vi "Manual Mode.vi"(0 "potent":dbl, 1 "Shooter":dbl, 2 "climb":bool, 3 "Button 1":bool, 5 "manual":bool) -> ()   [LabVIEW 2012]
uses:
  <vilib>/Rock Robotics/WPI/Solenoid/WPI_SolenoidValue.ctl
  <vilib>/Rock Robotics/WPI/Solenoid/WPI_SolenoidSetEnum.vi
  <vilib>/Rock Robotics/WPI/Joystick/WPI_JoystickGetSetRefNum.vi
  <vilib>/Rock Robotics/WPI/RobotDrive/WPI_RobotDriveArcadeDrive_Standard(NoSaturation).vi
  <vilib>/Rock Robotics/WPI/RobotDrive/WPI_RobotDriveGetSetRefNum.vi
panel:
  in  "Kick?":bool
  in  "Select":dbl(slide)=2.502610966057441 scale=0.3..4.1
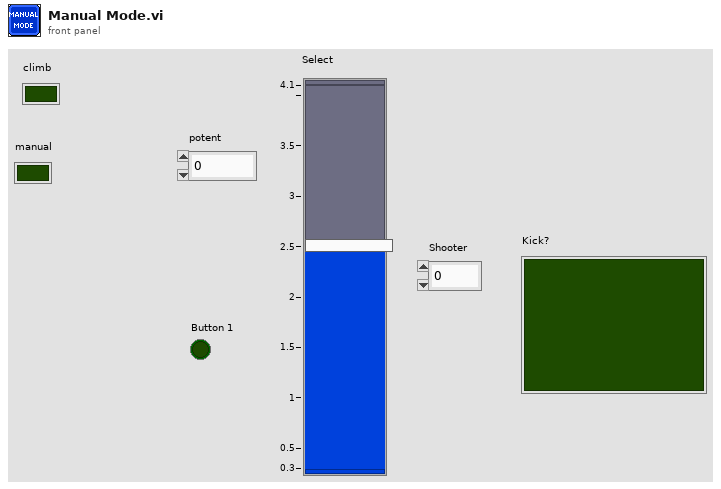
[diagram p1: front panel]
types:
  T1 = typedef "WPI_SolenoidValue.ctl" = enum16{"Off", "On", "Forward", "Reverse"}
  T2 = typedef "WPI_JoystickDevRef.ctl" = cluster{"Device":T3}
  T3 = typedef "WPI_JoystickDeviceEnum.ctl" = enum16{"USB 1", "USB 2", "USB 3", "USB 4", "Kinect 1", "Kinect 2"}
  T4 = typedef "WPI_JoystickButtonState.ctl" = cluster{"Button 1":bool, "Button 2":bool, "Button 3":bool, "Button 4":bool, "Button 5":bool, "Button 6":bool, "Button 7":bool, "Button 8":bool, "Button 9":bool, "Button 10":bool, "Button 11":bool, "Button 12":bool}
  T5 = typedef "WPI_MotorControlDeviceRef.ctl" = cluster{"DeviceStatus":errorcluster, "Type":enum16{"PWM", "CAN"}, "PWM":cluster{"Digital Module":T6, "PWM Channel":T7, "DeadBand":T8}, "CAN":cluster{"Device Number":u8, "Control Mode":T9, "Semaphore":T10, "Max Vout":dbl}, "Invert":bool, "TransformRef":T11, "InvTransformRef":T11}
  T6 = typedef "FPGA_TypedefDigitalModule.ctl" = enum16{"Digital Module 1", "Digital Module 2"}
  T7 = typedef "FPGA_DIOPWMChannel.ctl" = enum8{"PWM 1", "PWM 2", "PWM 3", "PWM 4", "PWM 5", "PWM 6", "PWM 7", "PWM 8", "PWM 9", "PWM 10", "Invalid"}
  T8 = typedef "WPI_PWMDeadband.ctl" = cluster{"Name":string, "maxPositivePwm":i32, "minPositivePwm":i32, "centerPwm":i32, "maxNegativePwm":i32, "minNegativePwm":i32, "angularRange":u16}
  T9 = typedef "WPI_CANJaguar_ControlMode.ctl" = enum8{"Percent VBus", "Current", "Speed", "Position", "Voltage"}
  T10 = typedef "Semaphore RefNum" = refnum<k1>
  T11 = typedef "WPI_PWMTransform_ConPane.ctl" = refnum<vi>
  T12 = typedef "WPI_SolenoidDevRef.ctl" = cluster{"DevStatus":errorcluster, "Solenoid Module":T13, "Forward Solenoid Channel":T14, "Reverse Solenoid Channel":T14}
  T13 = typedef "FPGA_TypedefSolenoidModule.ctl" = enum16{"Solenoid Module 1", "Solenoid Module 2"}
  T14 = typedef "WPI_SolenoidChannel.ctl" = enum8{"Solenoid 1", "Solenoid 2", "Solenoid 3", "Solenoid 4", "Solenoid 5", "Solenoid 6", "Solenoid 7", "Solenoid 8", "Invalid"}
  T15 = typedef "WPI_RobotDriveDevRef.ctl" = cluster{"DevStatus":errorcluster, "Motors[]":T5[], "Square Inputs":bool, "Max Output":dbl, "Isochronous":bool}
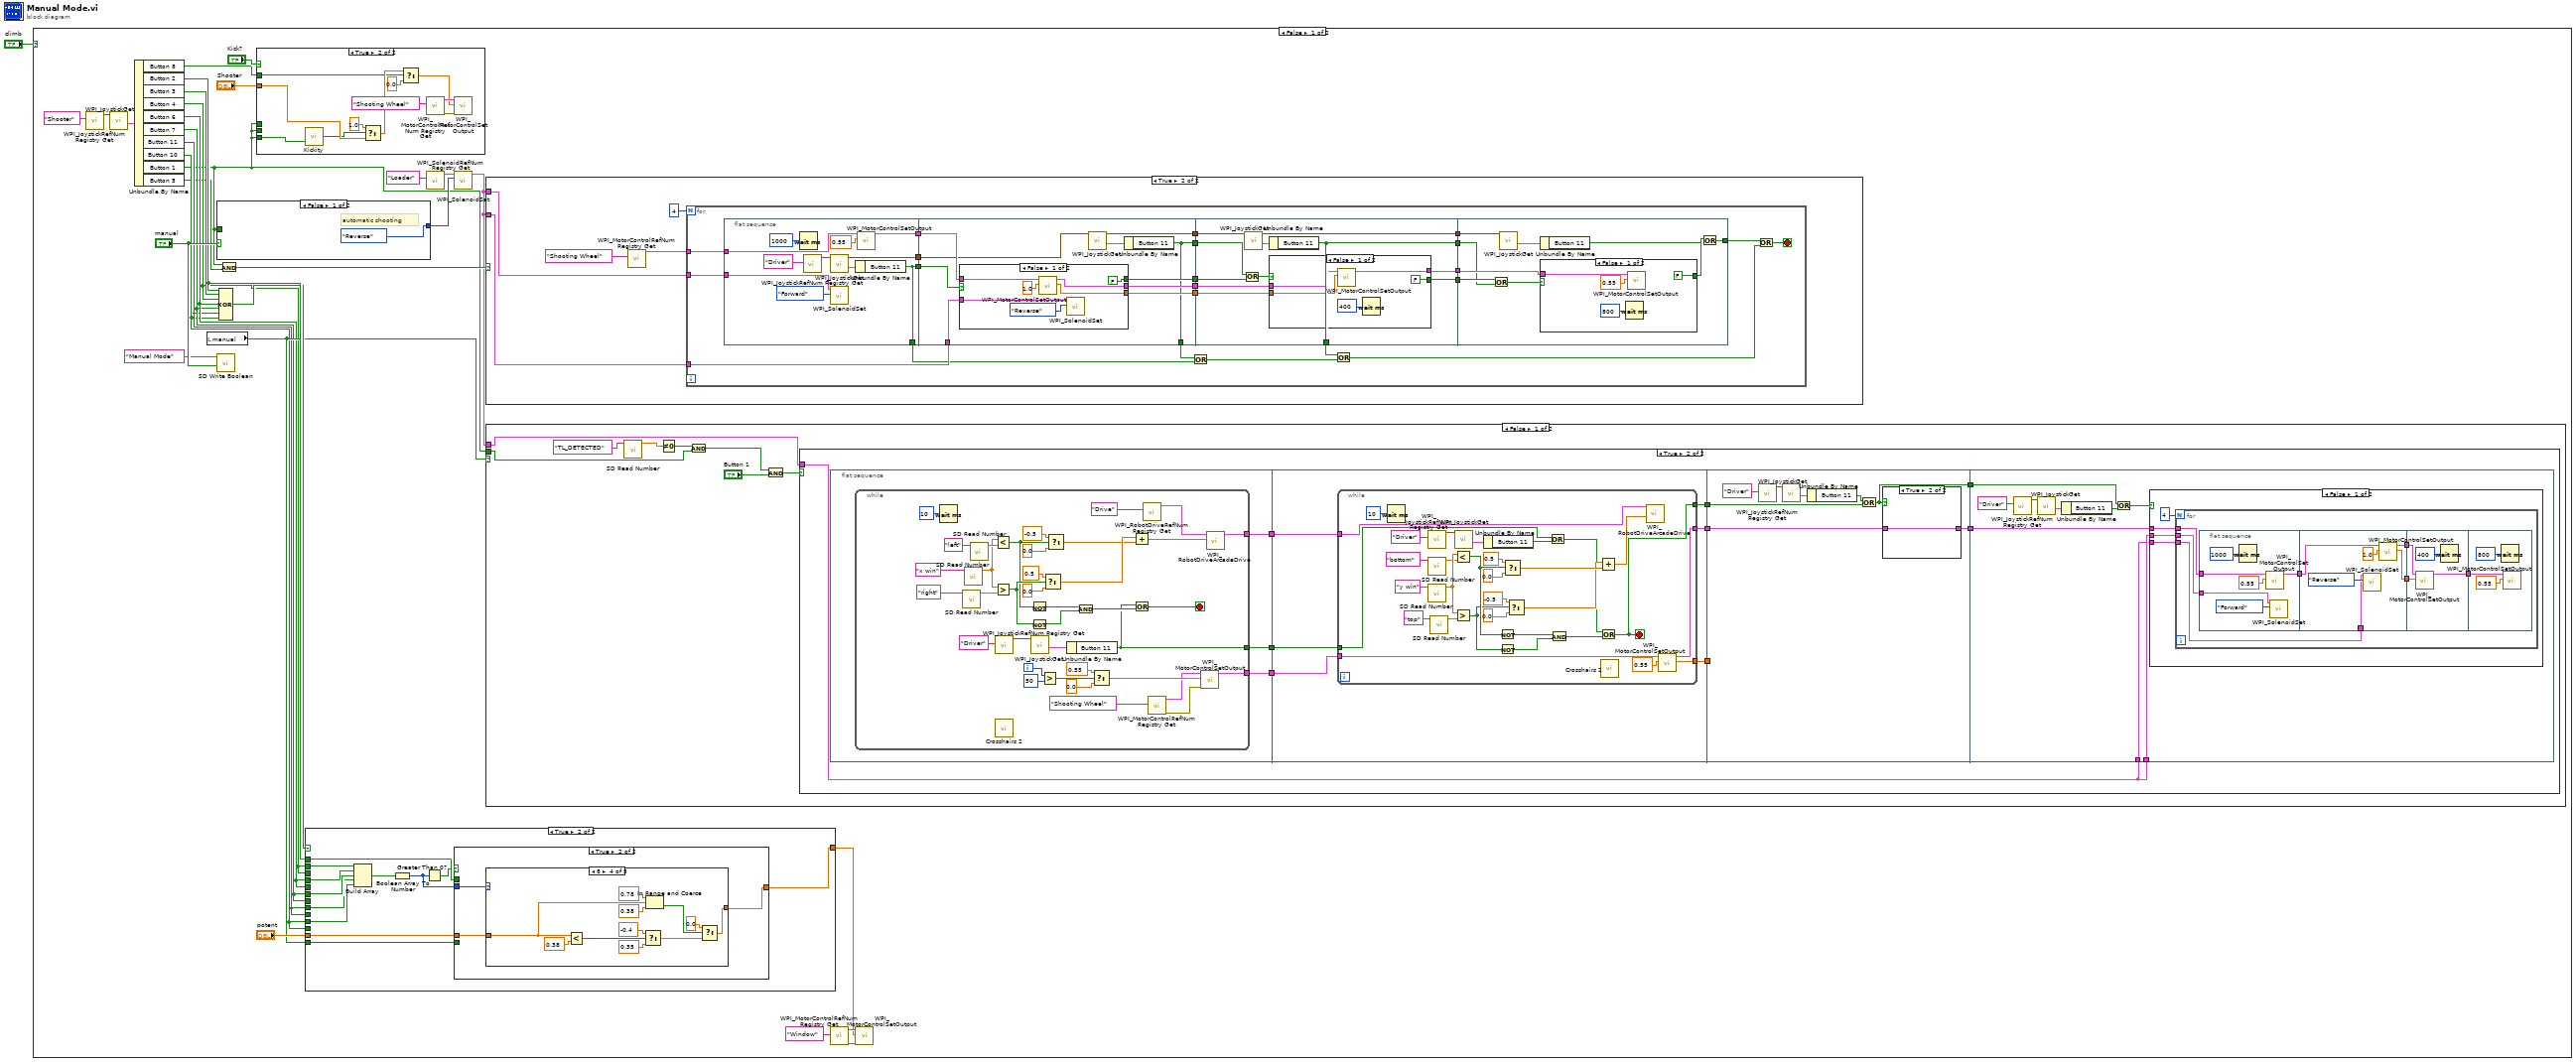
[diagram p0: block diagram]
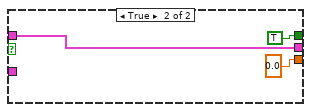
[diagram p3: hidden frame]
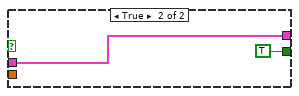
[diagram p4: hidden frame]
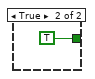
[diagram p5: hidden frame]
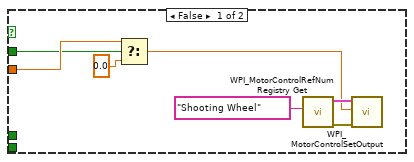
[diagram p6: hidden frame]
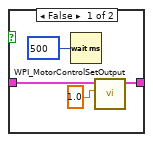
[diagram p8: hidden frame]
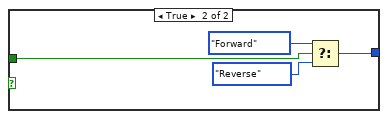
[diagram p11: hidden frame]
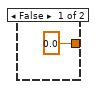
[diagram p12: hidden frame]
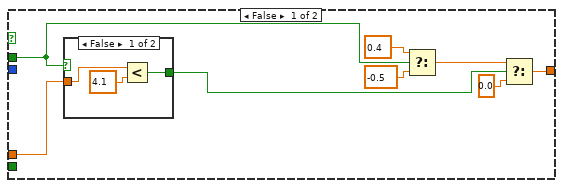
[diagram p13: hidden frame]
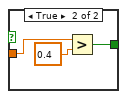
[diagram p14: hidden frame]
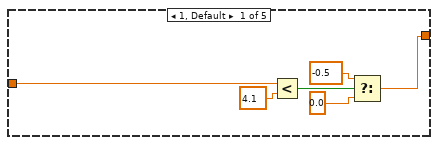
[diagram p15: hidden frame]
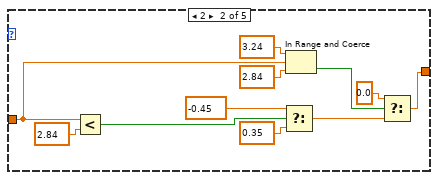
[diagram p16: hidden frame]
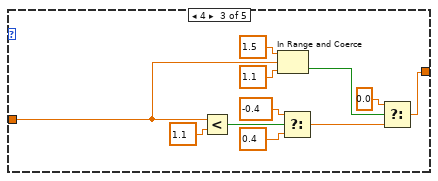
[diagram p17: hidden frame]
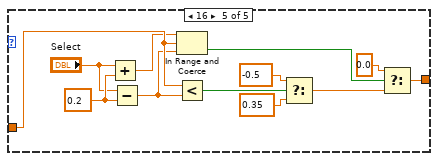
[diagram p18: hidden frame]
diagram:
  n1 = case shown="False" "climb" {
    frame False {
      n2 = call <vilib>:"WPI_JoystickRefNum Registry Get.vi"("refnum name"="Shooter") -> ("JoystickDevRef"=w30:T2)  [unwired: 9 in, 1 out]
      n3 = call <vilib>:"WPI_JoystickGet.vi"("JoystickDevRef"=w30) -> ("Buttons"=w28:T4)  [unwired: 4 in, 2 out]
      n4 = Unbundle By Name(w28) -> ("Button 8"=w15:bool, "Button 2"=w14:bool, "Button 3"=w13:bool, "Button 4"=w10:bool, "Button 6"=w9:bool, "Button 7"=w8:bool, "Button 11"=w7:bool, "Button 10"=w6:bool, "Button 1"=w2:bool, "Button 5"=w4:bool)
      n5 = local read "manual"() -> (w11:bool)
      n6 = case shown="False" "manual" {
        tunnel: w2 -> [_ w289]
        tunnel: [WPI_SolenoidValue."Reverse" ("Value") w286] -> w20
        frame False {
          # "automatic shooting"
        }
        frame True {
          n7 = Select(t=WPI_SolenoidValue."Forward" ("Value"), s=w289, f=WPI_SolenoidValue."Reverse" ("Value")) -> (s? t:f=w286:T1)
        }
      }
      n8 = call <vilib>:"SD Write Boolean.vi"("Boolean"="manual", "Name"="Manual Mode") -> ()  [unwired: 8 in, 2 out]
      n9 = Compound Arithmetic op=XOR(w14, w13, w10, w9, w8, w7, w6) -> (w12:bool)
      n10 = And(x=w2, y=w4) -> (x .and. y?=w5:bool)
      n11 = case shown="True" "Kick?" {
        tunnel: "Shooter" -> [w122 w131]
        tunnel: w15 -> [w121 w130]
        tunnel: w2 -> [_ _]
        tunnel: w2 -> [_ _]
        tunnel: w2 -> [_ w128]
        frame False {
          n12 = Select(t=w122, s=w121, f=0.0) -> (s? t:f=w124:dbl)
          n13 = call <vilib>:"WPI_MotorControlRefNum Registry Get.vi"("refnum name"="Shooting Wheel") -> ("error out"=w127:errorcluster, "MotorControlDevRef"=w125:T5)  [unwired: 9 in]
          n14 = call <vilib>:"WPI_MotorControlSetOutput.vi"("error in (no error)"=w127, "Output"=w124, "MotorControlDevRef"=w125) -> ()  [unwired: 6 in, 3 out]
        }
        frame True {
          n15 = call "Kickity.vi"("btn 1"=w128) -> ("kick"=w129:bool)  [unwired: 1 in]
          n16 = Select(t=1.0, s=w129, f=w131) -> (s? t:f=w133:dbl)
          n17 = Select(t=w133, s=w130, f=0.0) -> (s? t:f=w135:dbl)
          n18 = call <vilib>:"WPI_MotorControlRefNum Registry Get.vi"("refnum name"="Shooting Wheel") -> ("error out"=w138:errorcluster, "MotorControlDevRef"=w136:T5)  [unwired: 9 in]
          n19 = call <vilib>:"WPI_MotorControlSetOutput.vi"("error in (no error)"=w138, "Output"=w135, "MotorControlDevRef"=w136) -> ()  [unwired: 6 in, 3 out]
        }
      }
      n20 = case shown="True" w12 {
        tunnel: "potent" -> [_ w302]
        tunnel: [0.0 ("f") w301] -> w24
        tunnel: w14 -> [_ w300]
        tunnel: w11 -> [_ w299]
        tunnel: w10 -> [_ _]
        tunnel: w9 -> [_ _]
        tunnel: w8 -> [_ _]
        tunnel: w7 -> [_ _]
        tunnel: w6 -> [_ _]
        tunnel: w10 -> [_ w297]
        tunnel: w9 -> [_ w296]
        tunnel: w8 -> [_ w295]
        tunnel: w7 -> [_ w294]
        tunnel: w6 -> [_ w293]
        frame False {
        }
        frame True {
          n21 = Build Array(w297, w296, w295, w294, w293) -> (w298:bool[])
          n22 = Boolean Array To Number(Boolean array=w298) -> (number=w291:u32)
          n23 = Greater Than 0?(x=w291) -> (x > 0?=w292:bool)
          n24 = case shown="True" w292 {
            tunnel: w302 -> [w305 w319]
            tunnel: [w308 w318] -> w301
            tunnel: w300 -> [w306 _]
            tunnel: w291 -> [_ w317]
            tunnel: w299 -> [_ _]
            frame False {
              n25 = case shown="False" w306 {
                tunnel: w305 -> [w313 w316]
                tunnel: [w312 w314] -> w303
                frame False {
                  n26 = Less?(x=w313, y=4.1) -> (x < y?=w312:bool)
                }
                frame True {
                  n27 = Greater?(x=w316, y=0.4) -> (0:w314:bool)
                }
              }
              n28 = Select(t=0.4, s=w306, f=-0.5) -> (s? t:f=w304:dbl)
              n29 = Select(t=w304, s=w303, f=0.0) -> (s? t:f=w308:dbl)
            }
            frame True {
              n30 = case shown="8" w317 {
                tunnel: w319 -> [w325 w330 w339 w349 w363]
                tunnel: [w320 w334 w338 w350 w365] -> w318
                frame 1, Default {
                  n31 = Less?(x=w325, y=4.1) -> (x < y?=w323:bool)
                  n32 = Select(t=-0.5, s=w323, f=0.0) -> (s? t:f=w320:dbl)
                }
                frame 2 {
                  n33 = Less?(x=w330, y=2.84) -> (x < y?=w331:bool)
                  n34 = Select(t=-0.45, s=w331, f=0.35) -> (s? t:f=w335:dbl)
                  n35 = In Range and Coerce(upper limit=3.24, x=w330, lower limit=2.84) -> (In Range?=w336:bool)  [unwired: 1 out]
                  n36 = Select(t=0.0, s=w336, f=w335) -> (s? t:f=w334:dbl)
                }
                frame 4 {
                  n37 = Less?(x=w339, y=1.1) -> (x < y?=w343:bool)
                  n38 = In Range and Coerce(upper limit=1.5, x=w339, lower limit=1.1) -> (In Range?=w347:bool)  [unwired: 1 out]
                  n39 = Select(t=-0.4, s=w343, f=0.4) -> (s? t:f=w346:dbl)
                  n40 = Select(t=0.0, s=w347, f=w346) -> (s? t:f=w338:dbl)
                }
                frame 8 {
                  n41 = Less?(x=w349, y=0.38) -> (x < y?=w354:bool)
                  n42 = Select(t=-0.4, s=w354, f=0.35) -> (s? t:f=w357:dbl)
                  n43 = In Range and Coerce(upper limit=0.78, x=w349, lower limit=0.38) -> (In Range?=w358:bool)  [unwired: 1 out]
                  n44 = Select(t=0.0, s=w358, f=w357) -> (s? t:f=w350:dbl)
                }
                frame 16 {
                  w361 = 0.2 ("y")
                  n45 = Add(x="Select", y=w361) -> (x+y=w362:dbl)
                  n46 = Subtract(x="Select", y=w361) -> (x-y=w359:dbl)
                  n47 = In Range and Coerce(upper limit=w362, x=w363, lower limit=w359) -> (In Range?=w370:bool)  [unwired: 1 out]
                  n48 = Less?(x=w363, y=w359) -> (x < y?=w366:bool)
                  n49 = Select(t=-0.5, s=w366, f=0.35) -> (s? t:f=w369:dbl)
                  n50 = Select(t=0.0, s=w370, f=w369) -> (s? t:f=w365:dbl)
                }
              }
            }
          }
        }
      }
      n51 = call <vilib>:"WPI_SolenoidRefNum Registry Get.vi"("refnum name"="Loader") -> ("SolenoidDevRef"=w21:T12)  [unwired: 9 in, 1 out]
      n52 = call-poly <vilib>:"WPI_SolenoidSet.vi"("Value"=w20, "SolenoidDevRef"=w21) -> ("SolenoidDevRef"=w3:T12)  [unwired: 8 in, 1 out]
      n53 = case shown="True" w5 {
        tunnel: w3 -> [_ w34]
        tunnel: w3 -> [_ w33]
        frame False {
        }
        frame True {
          n54 = call <vilib>:"WPI_MotorControlRefNum Registry Get.vi"("refnum name"="Shooting Wheel") -> ("MotorControlDevRef"=w31:T5)  [unwired: 9 in, 1 out]
          n55 = for {
            N: 4 -> [_]
            tunnel: w34 -> [w53]
            tunnel: w33 -> [w52]
            tunnel: w31 -> [w51]
            stop <- w42 stop-if-true
            n56 = flat-sequence {
              tunnel: [w60] -> w56
              tunnel: [w58] -> w50
              tunnel: [w59] -> w41
              tunnel: [w59] -> w36
              tunnel: w51 -> [w65]
              tunnel: w53 -> [w66]
              tunnel: [w78] -> w57
              tunnel: w56 -> [w77]
              tunnel: [w76] -> w55
              tunnel: w52 -> [w75]
              tunnel: w50 -> [w73]
              tunnel: [w72] -> w49
              tunnel: [w70] -> w47
              tunnel: w41 -> [w69]
              tunnel: [w71] -> w40
              tunnel: [w70] -> w39
              tunnel: w57 -> [w99]
              tunnel: w55 -> [w98]
              tunnel: [w97] -> w54
              tunnel: w49 -> [w95]
              tunnel: [w94] -> w48
              tunnel: [w89] -> w45
              tunnel: w40 -> [w93]
              tunnel: w39 -> [w92]
              tunnel: [w90] -> w38
              tunnel: [w89] -> w37
              tunnel: w54 -> [w115]
              tunnel: w48 -> [w113]
              tunnel: [w107] -> w43
              tunnel: w38 -> [w112]
              tunnel: w37 -> [w111]
              frame #0 {
                n57 = Wait (ms)(milliseconds to wait=u32 1000) -> ()  [unwired: 1 out]
                n58 = call <vilib>:"WPI_JoystickRefNum Registry Get.vi"("refnum name"="Driver") -> ("JoystickDevRef"=w64:T2)  [unwired: 9 in, 1 out]
                n59 = call <vilib>:"WPI_JoystickGet.vi"("JoystickDevRef"=w64) -> ("Buttons"=w63:T4, "JoystickDevRef"=w58:T2)  [unwired: 4 in, 1 out]
                n60 = call-poly <vilib>:"WPI_SolenoidSet.vi"("Value"=WPI_SolenoidValue."Forward", "SolenoidDevRef"=w66) -> ()  [unwired: 8 in, 2 out]
                n61 = Unbundle By Name(w63) -> ("Button 11"=w59:bool)
                n62 = call <vilib>:"WPI_MotorControlSetOutput.vi"("Output"=0.55, "MotorControlDevRef"=w65) -> ("MotorControlDevRef"=w60:T5)  [unwired: 7 in, 2 out]
              }
              frame #1 {
                n63 = case shown="False" w69 {
                  tunnel: [w84 0.0 ("Motor Output")] -> w78
                  tunnel: w77 -> [w83 w87]
                  tunnel: [w82 w87] -> w76
                  tunnel: w75 -> [w80 _]
                  tunnel: [FALSE TRUE] -> w71
                  frame False {
                    n64 = call <vilib>:"WPI_MotorControlSetOutput.vi"("Output"=1.0, "MotorControlDevRef"=w83) -> ("Motor Output"=w84:dbl, "MotorControlDevRef"=w82:T5)  [unwired: 7 in, 1 out]
                    n65 = call-poly <vilib>:"WPI_SolenoidSet.vi"("Value"=WPI_SolenoidValue."Reverse", "SolenoidDevRef"=w80) -> ()  [unwired: 8 in, 2 out]
                  }
                  frame True {
                  }
                }
                n66 = call <vilib>:"WPI_JoystickGet.vi"("JoystickDevRef"=w73) -> ("Buttons"=w74:T4, "JoystickDevRef"=w72:T2)  [unwired: 4 in, 1 out]
                n67 = Unbundle By Name(w74) -> ("Button 11"=w70:bool)
              }
              frame #2 {
                n68 = Or(x=w92, y=w93) -> (x .or. y?=w91:bool)
                n69 = call <vilib>:"WPI_JoystickGet.vi"("JoystickDevRef"=w95) -> ("Buttons"=w96:T4, "JoystickDevRef"=w94:T2)  [unwired: 4 in, 1 out]
                n70 = Unbundle By Name(w96) -> ("Button 11"=w89:bool)
                n71 = case shown="False" w91 {
                  tunnel: w99 -> [w103 _]
                  tunnel: w98 -> [w102 w105]
                  tunnel: [w101 w105] -> w97
                  tunnel: [FALSE TRUE] -> w90
                  frame False {
                    n72 = call <vilib>:"WPI_MotorControlSetOutput.vi"("Output"=w103, "MotorControlDevRef"=w102) -> ("MotorControlDevRef"=w101:T5)  [unwired: 7 in, 2 out]
                    n73 = Wait (ms)(milliseconds to wait=u32 400) -> ()  [unwired: 1 out]
                  }
                  frame True {
                  }
                }
              }
              frame #3 {
                n74 = Or(x=w112, y=w111) -> (x .or. y?=w110:bool)
                n75 = call <vilib>:"WPI_JoystickGet.vi"("JoystickDevRef"=w113) -> ("Buttons"=w114:T4)  [unwired: 4 in, 2 out]
                n76 = Unbundle By Name(w114) -> ("Button 11"=w108:bool)
                n77 = case shown="False" w110 {
                  tunnel: w115 -> [w119 _]
                  tunnel: [FALSE TRUE] -> w109
                  frame False {
                    n78 = Wait (ms)(milliseconds to wait=u32 800) -> ()  [unwired: 1 out]
                    n79 = call <vilib>:"WPI_MotorControlSetOutput.vi"("Output"=0.55, "MotorControlDevRef"=w119) -> ()  [unwired: 7 in, 3 out]
                  }
                  frame True {
                  }
                }
                n80 = Or(x=w109, y=w108) -> (x .or. y?=w107:bool)
              }
            }
            n81 = Or(x=w47, y=w36) -> (x .or. y?=w46:bool)
            n82 = Or(x=w45, y=w46) -> (x .or. y?=w44:bool)
            n83 = Or(x=w43, y=w44) -> (x .or. y?=w42:bool)
          }
        }
      }
      n84 = case shown="False" w11 {
        tunnel: w3 -> [w140 _]
        tunnel: w2 -> [w139 _]
        frame False {
          n85 = call <vilib>:"SD Read Number.vi"("Name"="TL_DETECTED") -> ("Numeric"=w141:dbl)  [unwired: 8 in, 2 out]
          n86 = Not Equal To 0?(x=w141) -> (x != 0?=w142:bool)
          n87 = And(x=w142, y=w139) -> (x .and. y?=w144:bool)
          n88 = And(x=w144, y="Button 1") -> (x .and. y?=w146:bool)
          n89 = case shown="True" w146 {
            tunnel: w140 -> [_ w150]
            frame False {
            }
            frame True {
              n90 = flat-sequence {
                tunnel: [w158] -> w155
                tunnel: [w157] -> w154
                tunnel: [w156] -> w149
                tunnel: w155 -> [w201]
                tunnel: w154 -> [w200]
                tunnel: [w199] -> w153
                tunnel: [w198] -> w152
                tunnel: w149 -> [w197]
                tunnel: [w196] -> w148
                tunnel: [w235] -> w151
                tunnel: w153 -> [w236]
                tunnel: w152 -> [_]
                tunnel: w148 -> [w234]
                tunnel: [w233] -> w147
                tunnel: w151 -> [w254]
                tunnel: w150 -> [w253]
                tunnel: w150 -> [w252]
                tunnel: w147 -> [w247]
                frame #0 {
                  n91 = while {
                    tunnel: [w183] -> w158
                    tunnel: [w172] -> w157
                    tunnel: [w159] -> w156
                    i -> [w189]
                    stop <- w160 stop-if-true
                    n92 = Wait (ms)(milliseconds to wait=u32 10) -> ()  [unwired: 1 out]
                    n93 = call <vilib>:"SD Read Number.vi"("Name"="right") -> ("Numeric"=w179:dbl)  [unwired: 8 in, 2 out]
                    n94 = call <vilib>:"SD Read Number.vi"("Name"="x win") -> ("Numeric"=w177:dbl)  [unwired: 8 in, 2 out]
                    n95 = call <vilib>:"SD Read Number.vi"("Name"="left") -> ("Numeric"=w178:dbl)  [unwired: 8 in, 2 out]
                    n96 = Less?(x=w177, y=w178) -> (x < y?=w168:bool)
                    n97 = Greater?(x=w177, y=w179) -> (0:w169:bool)
                    n98 = call <vilib>:"WPI_JoystickRefNum Registry Get.vi"("refnum name"="Driver") -> ("JoystickDevRef"=w164:T2)  [unwired: 9 in, 1 out]
                    n99 = call "Crosshairs 2.vi"() -> ()  [unwired: 2 in]
                    n100 = Not(x=w168) -> (.not. x?=w171:bool)
                    n101 = Not(x=w169) -> (.not. x?=w170:bool)
                    n102 = call <vilib>:"WPI_JoystickGet.vi"("JoystickDevRef"=w164) -> ("Buttons"=w163:T4)  [unwired: 4 in, 2 out]
                    n103 = Greater?(x=w189, y=50) -> (0:w187:bool)
                    n104 = Select(t=0.5, s=w169, f=0.0) -> (s? t:f=w167:dbl)
                    n105 = Select(t=-0.5, s=w168, f=0.0) -> (s? t:f=w166:dbl)
                    n106 = Unbundle By Name(w163) -> ("Button 11"=w159:bool)
                    n107 = And(x=w171, y=w170) -> (x .and. y?=w161:bool)
                    n108 = Select(t=0.55, s=w187, f=0.0) -> (s? t:f=w190:dbl)
                    n109 = Add(x=w167, y=w166) -> (x+y=w165:dbl)
                    n110 = Or(x=w159, y=w161) -> (x .or. y?=w160:bool)
                    n111 = call <vilib>:"WPI_RobotDriveRefNum Registry Get.vi"("refnum name"="Drive") -> ("RobotDriveDevRef"=w194:T15)  [unwired: 9 in, 1 out]
                    n112 = call <vilib>:"WPI_MotorControlRefNum Registry Get.vi"("refnum name"="Shooting Wheel") -> ("error out"=w192:errorcluster, "MotorControlDevRef"=w184:T5)  [unwired: 9 in]
                    n113 = call <vilib>:"WPI_MotorControlSetOutput.vi"("error in (no error)"=w192, "Output"=w190, "MotorControlDevRef"=w184) -> ("MotorControlDevRef"=w183:T5)  [unwired: 6 in, 2 out]
                    n114 = call-poly <vilib>:"WPI_RobotDriveArcadeDrive.vi"("X axis value"=w165, "RobotDriveDevRef"=w194) -> ("RobotDriveDevRef"=w172:T15)  [unwired: 7 in, 2 out]
                  }
                }
                frame #1 {
                  n115 = while {
                    tunnel: w201 -> [w228]
                    tunnel: w200 -> [w227]
                    tunnel: [w215] -> w199
                    tunnel: [w214] -> w198
                    tunnel: w197 -> [w207]
                    tunnel: [w203] -> w196
                    stop <- w203 stop-if-true
                    n116 = Wait (ms)(milliseconds to wait=u32 10) -> ()  [unwired: 1 out]
                    n117 = call <vilib>:"SD Read Number.vi"("Name"="bottom") -> ("Numeric"=w224:dbl)  [unwired: 8 in, 2 out]
                    n118 = call <vilib>:"WPI_JoystickRefNum Registry Get.vi"("refnum name"="Driver") -> ("JoystickDevRef"=w210:T2)  [unwired: 9 in, 1 out]
                    n119 = call <vilib>:"SD Read Number.vi"("Name"="y win") -> ("Numeric"=w225:dbl)  [unwired: 8 in, 2 out]
                    n120 = call <vilib>:"SD Read Number.vi"("Name"="top") -> ("Numeric"=w226:dbl)  [unwired: 8 in, 2 out]
                    n121 = Less?(x=w225, y=w224) -> (x < y?=w217:bool)
                    n122 = Greater?(x=w225, y=w226) -> (0:w216:bool)
                    n123 = call <vilib>:"WPI_JoystickGet.vi"("JoystickDevRef"=w210) -> ("Buttons"=w209:T4)  [unwired: 4 in, 2 out]
                    n124 = Unbundle By Name(w209) -> ("Button 11"=w206:bool)
                    n125 = Not(x=w217) -> (.not. x?=w219:bool)
                    n126 = Not(x=w216) -> (.not. x?=w218:bool)
                    n127 = Select(t=0.5, s=w217, f=0.0) -> (s? t:f=w213:dbl)
                    n128 = Select(t=-0.5, s=w216, f=0.0) -> (s? t:f=w212:dbl)
                    n129 = Or(x=w207, y=w206) -> (x .or. y?=w205:bool)
                    n130 = And(x=w219, y=w218) -> (x .and. y?=w204:bool)
                    n131 = Add(x=w212, y=w213) -> (x+y=w211:dbl)
                    n132 = Or(x=w205, y=w204) -> (x .or. y?=w203:bool)
                    n133 = call "Crosshairs 2.vi"() -> ()  [unwired: 2 in]
                    n134 = call-poly <vilib>:"WPI_RobotDriveArcadeDrive.vi"("Y axis value"=w211, "RobotDriveDevRef"=w227) -> ()  [unwired: 7 in, 3 out]
                    n135 = call <vilib>:"WPI_MotorControlSetOutput.vi"("Output"=0.55, "MotorControlDevRef"=w228) -> ("Motor Output"=w214:dbl, "MotorControlDevRef"=w215:T5)  [unwired: 7 in, 1 out]
                  }
                }
                frame #2 {
                  n136 = call <vilib>:"WPI_JoystickRefNum Registry Get.vi"("refnum name"="Driver") -> ("JoystickDevRef"=w240:T2)  [unwired: 9 in, 1 out]
                  n137 = call <vilib>:"WPI_JoystickGet.vi"("JoystickDevRef"=w240) -> ("Buttons"=w239:T4)  [unwired: 4 in, 2 out]
                  n138 = Unbundle By Name(w239) -> ("Button 11"=w237:bool)
                  n139 = Or(x=w237, y=w234) -> (x .or. y?=w233:bool)
                  n140 = case shown="True" w233 {
                    tunnel: [w243 w245] -> w235
                    tunnel: w236 -> [w242 w245]
                    frame False {
                      n141 = Wait (ms)(milliseconds to wait=u32 500) -> ()  [unwired: 1 out]
                      n142 = call <vilib>:"WPI_MotorControlSetOutput.vi"("Output"=1.0, "MotorControlDevRef"=w242) -> ("MotorControlDevRef"=w243:T5)  [unwired: 7 in, 2 out]
                    }
                    frame True {
                    }
                  }
                }
                frame #3 {
                  n143 = call <vilib>:"WPI_JoystickRefNum Registry Get.vi"("refnum name"="Driver") -> ("JoystickDevRef"=w251:T2)  [unwired: 9 in, 1 out]
                  n144 = call <vilib>:"WPI_JoystickGet.vi"("JoystickDevRef"=w251) -> ("Buttons"=w250:T4)  [unwired: 4 in, 2 out]
                  n145 = Unbundle By Name(w250) -> ("Button 11"=w248:bool)
                  n146 = Or(x=w247, y=w248) -> (x .or. y?=w246:bool)
                  n147 = case shown="False" w246 {
                    tunnel: w254 -> [w257 _]
                    tunnel: w253 -> [w256 _]
                    tunnel: w252 -> [w255 _]
                    frame False {
                      n148 = for {
                        N: 4 -> [_]
                        tunnel: w257 -> [w261]
                        tunnel: w256 -> [w260]
                        tunnel: w255 -> [w259]
                        n149 = flat-sequence {
                          tunnel: [w266] -> w264
                          tunnel: w260 -> [w269]
                          tunnel: w261 -> [w270]
                          tunnel: [w276] -> w265
                          tunnel: w264 -> [w275]
                          tunnel: [w274] -> w263
                          tunnel: w259 -> [w272]
                          tunnel: w265 -> [w280]
                          tunnel: w263 -> [w279]
                          tunnel: [w278] -> w262
                          tunnel: w262 -> [w284]
                          frame #0 {
                            n150 = Wait (ms)(milliseconds to wait=u32 1000) -> ()  [unwired: 1 out]
                            n151 = call <vilib>:"WPI_MotorControlSetOutput.vi"("Output"=0.55, "MotorControlDevRef"=w270) -> ("MotorControlDevRef"=w266:T5)  [unwired: 7 in, 2 out]
                            n152 = call-poly <vilib>:"WPI_SolenoidSet.vi"("Value"=WPI_SolenoidValue."Forward", "SolenoidDevRef"=w269) -> ()  [unwired: 8 in, 2 out]
                          }
                          frame #1 {
                            n153 = call-poly <vilib>:"WPI_SolenoidSet.vi"("Value"=WPI_SolenoidValue."Reverse", "SolenoidDevRef"=w272) -> ()  [unwired: 8 in, 2 out]
                            n154 = call <vilib>:"WPI_MotorControlSetOutput.vi"("Output"=1.0, "MotorControlDevRef"=w275) -> ("Motor Output"=w276:dbl, "MotorControlDevRef"=w274:T5)  [unwired: 7 in, 1 out]
                          }
                          frame #2 {
                            n155 = call <vilib>:"WPI_MotorControlSetOutput.vi"("Output"=w280, "MotorControlDevRef"=w279) -> ("MotorControlDevRef"=w278:T5)  [unwired: 7 in, 2 out]
                            n156 = Wait (ms)(milliseconds to wait=u32 400) -> ()  [unwired: 1 out]
                          }
                          frame #3 {
                            n157 = Wait (ms)(milliseconds to wait=u32 800) -> ()  [unwired: 1 out]
                            n158 = call <vilib>:"WPI_MotorControlSetOutput.vi"("Output"=0.55, "MotorControlDevRef"=w284) -> ()  [unwired: 7 in, 3 out]
                          }
                        }
                      }
                    }
                    frame True {
                    }
                  }
                }
              }
            }
          }
        }
        frame True {
        }
      }
      n159 = call <vilib>:"WPI_MotorControlRefNum Registry Get.vi"("refnum name"="Window") -> ("error out"=w23:errorcluster, "MotorControlDevRef"=w25:T5)  [unwired: 9 in]
      n160 = call <vilib>:"WPI_MotorControlSetOutput.vi"("error in (no error)"=w23, "Output"=w24, "MotorControlDevRef"=w25) -> ()  [unwired: 6 in, 3 out]
    }
    frame True {
    }
  }
